vi "error control.vi"(8 "에러 입력(에러 없음)":errorcluster, 10 "Image Out":T2, 11 "참조 번호 입력":T1) -> (0 "에러 출력":errorcluster, 2 "New Image":T2, 3 "참조 번호 출력":T1)   [LabVIEW 2018]
uses:
  <vilib>/vision/Image Controls.llb/IMAQ Image.ctl
  <vilib>/userdefined/High Color/IMAQdx.ctl
  <vilib>/vision/driver/NI_Vision_Acquisition_Software.lvlib
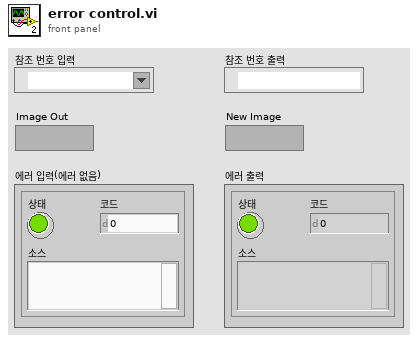
[diagram p1: front panel]
types:
  T1 = typedef "IMAQdx.ctl" = refnum<k21>
  T2 = typedef "IMAQ Image.ctl" = refnum<image>
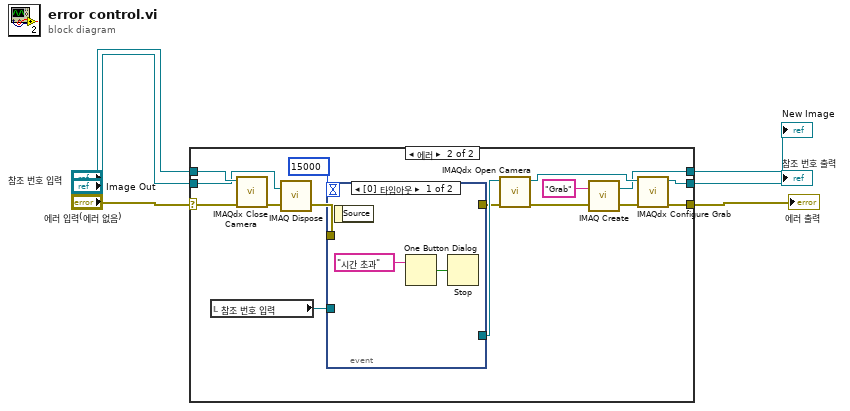
[diagram p0: block diagram]
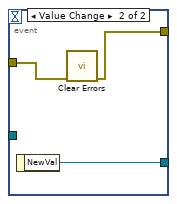
[diagram p3: hidden frame]
diagram:
  n1 = case shown="에러" "에러 입력(에러 없음)" {
    selector: "에러 입력(에러 없음)" -> [w9 w24]
    tunnel: [w9 w17] -> w6
    tunnel: "참조 번호 입력" -> [w8 w23]
    tunnel: [w8 w16] -> w2
    tunnel: "Image Out" -> [w7 w22]
    tunnel: [w7 w15] -> w4
    frame No Error {
    }
    frame Error {
      n2 = local read "참조 번호 입력"() -> (w12:T1)
      n3 = call <vilib>:"IMAQdx Close Camera.vi"("error in"=w24, "Session In"=w23) -> ("error out"=w25:errorcluster)  [unwired: 9 in]
      n4 = call "IMAQ Dispose"("Image"=w22, "error in (no error)"=w25) -> ("error out"=w13:errorcluster)  [unwired: 4 in]
      n5 = event shown="[0] 타임아웃" {
        selector: _ -> [_ _]
        dyn-events: _ -> [_ _]
        timeout: 15000 -> [_ _]
        tunnel: w13 -> [_ w29]
        tunnel: w12 -> [_ _]
        tunnel: [_ w30] -> w11
        tunnel: [_ w28] -> w10
        event Timeout {
          n6 = event-data() -> ()  [unwired: 1 in, 1 out]
          n7 = One Button Dialog(message="시간 초과" ("메시지")) -> (true=w26:bool)  [unwired: 1 in]
          n8 = Stop(stop? (T)=w26) -> ()
        }
        event Value Change {
          n9 = event-data() -> ("NewVal"=w30:T1)  [unwired: 1 in]
          n10 = call <vilib>:"Clear Errors.vi"("error in (no error)"=w29) -> ("error out"=w28:errorcluster)  [unwired: 5 in, 1 out]
        }
      }
      n11 = call <vilib>:"IMAQdx Open Camera.vi"("error in"=w10, "Session In"=w11) -> ("error out"=w20:errorcluster, "Session Out"=w19:T1)  [unwired: 8 in]
      n12 = call "IMAQ Create"("Image Name"="Grab", "error in (no error)"=w20) -> ("New Image"=w15:T2, "error out"=w18:errorcluster)  [unwired: 3 in]
      n13 = call <vilib>:"IMAQdx Configure Grab.vi"("error in"=w18, "Session In"=w19) -> ("error out"=w17:errorcluster, "Session Out"=w16:T1)  [unwired: 8 in]
    }
  }
  "에러 출력" <- w6
  "New Image" <- w4
  "참조 번호 출력" <- w2
